vi "Delete Stale Samples.vi"(8 "error in (no error)":errorcluster, 11 "buffer":refnum<data-value>) -> (0 "error out":errorcluster, 1 "new channel length":i32, 2 "new buffer timestamp":timestamp format="%<%H:%M:%S%6u\n%x>T", 3 "buffer":refnum<data-value>)   [LabVIEW 2017, in "Waveforms (N Ch).lvclass"]
uses:
  <vilib>/addons/_NISVFA/_Shared subVIs/Data Objects/Waveforms (DBL)/Waveforms (N Ch).lvclass
  C:/Program Files (x86)/National Instruments/LabVIEW 2017/vi.lib/addons/_NISVFA/_Shared subVIs/Data Objects/Data/Data.lvclass
  <vilib>/addons/_NISVFA/_Shared subVIs/Data Objects/Data/Data.lvclass/Data.ctl
  <vilib>/addons/_NISVFA/_Shared subVIs/Data Objects/Waveforms (DBL)/Waveforms (N Ch).lvclass/Waveforms (N Ch).ctl
  <vilib>/addons/_NISVFA/_Shared subVIs/Common/svc_Get Waveform Subset (Index).vi
  <vilib>/addons/_NISVFA/_Shared subVIs/Common/sv_Get NI Property Name String.vi
  <vilib>/addons/_NISVFA/_Shared subVIs/Common/svc_Get Array Subset (Index).vi
  <vilib>/addons/_NISVFA/_Shared subVIs/Common/svc_Coerce Index and Length.vi
  <vilib>/addons/_NISVFA/_Shared subVIs/Common/svc_Conditional Merge Error.vi
  <vilib>/addons/_NISVFA/_Shared subVIs/Data Objects/Data/Data.lvclass
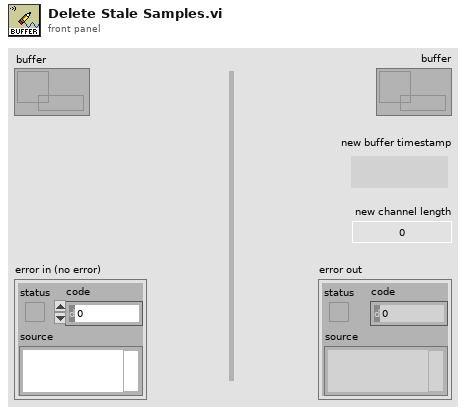
[diagram p1: front panel]
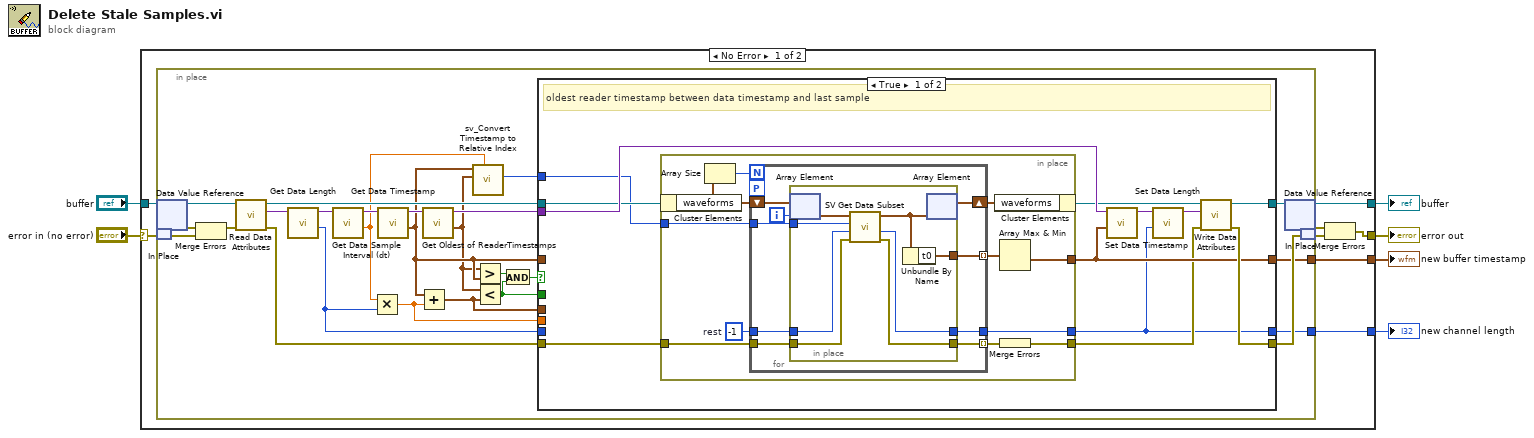
[diagram p0: block diagram]
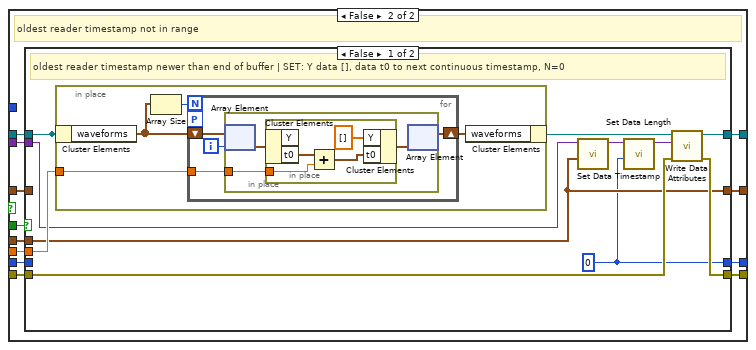
[diagram p2: hidden frame]
diagram:
  n1 = case shown="No Error" "error in (no error)" {
    selector: "error in (no error)" -> [w12 w122]
    tunnel: [w9 w122] -> w5
    tunnel: [w14 w123] -> w3
    tunnel: "buffer" -> [w13 w123]
    tunnel: [w8 _] -> w2
    tunnel: [w7 _] -> w1
    frame No Error {
      n2 = in-place {
        in-place-border: [w21] -> w8
        in-place-border: [w20] -> w7
        n3 = in-place-dvr #1(w13) -> (w39:refnum<class "Waveforms (N Ch).lvclass">, w38:errorcluster)
        n4 = in-place-match #2(w12) -> (w37:errorcluster)
        n5 = Merge Errors(w38, w37) -> (w36:errorcluster)
        n6 = call <vilib>:"Read Data Attributes.vi"("error in (no error)"=w36, "Data in"=w39) -> ("error out"=w34:errorcluster, "data attributes"=w28:variant, "Data out"=w35:refnum<class "Waveforms (N Ch).lvclass">)  [unwired: 7 in]
        n7 = call <vilib>:"Get Data Length.vi"("variant in"=w28) -> ("number of samples"=w19:i32, "variant out"=w29:variant)  [unwired: 9 in]
        n8 = call <vilib>:"Get Data Sample Interval (dt).vi"("variant in"=w29) -> ("dt [s]"=w18:dbl, "variant out"=w27:variant)  [unwired: 9 in]
        n9 = Multiply(x=w18, y=w19) -> (x*y=w22:dbl)
        n10 = call <vilib>:"Get Data Timestamp.vi"("variant in"=w27) -> ("timestamp"=w17:timestamp, "variant out"=w30:variant)  [unwired: 9 in]
        n11 = Add(x=w17, y=w22) -> (x+y=w23:timestamp)
        n12 = call <vilib>:"Get Oldest of ReaderTimestamps.vi"("data attributes"=w30) -> ("timestamp"=w16:timestamp, "data attributes"=w33:variant)  [unwired: 8 in, 1 out]
        n13 = call <vilib>:"sv_Convert Timestamp to Relative Index.vi"("waveform dt"=w18, "timestamp"=w16, "waveform timestamp"=w17) -> ("Y index"=w15:i32)  [unwired: 8 in]
        n14 = Greater?(x=w16, y=w17) -> (0:w25:bool)
        n15 = Less?(x=w16, y=w23) -> (x < y?=w24:bool)
        n16 = And(x=w25, y=w24) -> (x .and. y?=w26:bool)
        n17 = case shown="True" w26 {
          tunnel: w35 -> [w46 w88]
          tunnel: w34 -> [w43 w87]
          tunnel: w33 -> [w47 w91]
          tunnel: [w51 w90] -> w32
          tunnel: [w50 w89] -> w31
          tunnel: w24 -> [_ w86]
          tunnel: w23 -> [_ w85]
          tunnel: w22 -> [_ w84]
          tunnel: [w45 w83] -> w21
          tunnel: [w42 w82] -> w20
          tunnel: w17 -> [_ w81]
          tunnel: w19 -> [_ w80]
          tunnel: w15 -> [w40 _]
          frame True {
            # "oldest reader timestamp between data timestamp and last sample"
            n18 = in-place {
              in-place-border: w43 -> [w62]
              in-place-border: [w60] -> w45
              in-place-border: [w59] -> w44
              in-place-border: [w58] -> w42
              in-place-border: w40 -> [w56]
              w52 = -1  # rest
              n19 = in-place-cluster #3(w46) -> ("waveforms"=w53:waveform(dbl)[])
              n20 = Array Size(array=w53) -> (size(s)=w54:i32)
              n21 = for {
                N: w54 -> [_]
                tunnel: w62 -> [w71]
                tunnel: [w70] -> w57 mode=indexing
                tunnel: [w69] -> w61 mode=indexing
                workers-P: _ -> [_]
                tunnel: [w68] -> w58
                tunnel: w56 -> [w67]
                shift-right: [w64] -> w55
                shift-left: w53 -> [w66]
                tunnel: w52 -> [w63]
                i -> [w65]
                n22 = in-place {
                  in-place-border: w71 -> [w79]
                  in-place-border: [w78] -> w70
                  in-place-border: [w77] -> w69
                  in-place-border: [w76] -> w68
                  in-place-border: w67 -> [w75]
                  in-place-border: w63 -> [w72]
                  n23 = in-place-array #4(w66, w65) -> (w74:waveform(dbl))
                  n24 = call-poly <vilib>:"SV Get Data Subset.vi"("error in (no error)"=w79, "length (-1 = all)"=w72, "start index (0)"=w75, "waveform in"=w74) -> ("error out"=w78:errorcluster, "actual length"=w76:i32, "waveform subset"=w73:waveform(dbl))  [unwired: 2 in, 3 out]
                  n25 = Unbundle By Name(w73) -> ("t0"=w77:timestamp)
                  n26 = in-place-array #4(w73) -> (w64:waveform(dbl)[])  [unwired: 1 out]
                }
              }
              n27 = in-place-cluster #3("waveforms"=w55) -> (w41:refnum<class "Waveforms (N Ch).lvclass">)
              n28 = Array Max & Min(array=w61) -> (min value=w60:timestamp)  [unwired: 3 out]
              n29 = Merge Errors(w57) -> (w59:errorcluster)
            }
            n30 = call <vilib>:"Set Data Timestamp.vi"("timestamp"=w45, "variant in"=w47) -> ("variant out"=w49:variant)  [unwired: 9 in]
            n31 = call <vilib>:"Set Data Length.vi"("number of samples"=w42, "variant in"=w49) -> ("variant out"=w48:variant)  [unwired: 9 in]
            n32 = call <vilib>:"Write Data Attributes.vi"("error in (no error)"=w44, "data attributes"=w48, "Data in"=w41) -> ("error out"=w50:errorcluster, "Data out"=w51:refnum<class "Waveforms (N Ch).lvclass">)  [unwired: 7 in]
          }
          frame False {
            # "oldest reader timestamp not in range"
            n33 = case shown="False" w86 {
              tunnel: [w102 w121] -> w89
              tunnel: [w94 w120] -> _
              tunnel: [w101 w120] -> w90
              tunnel: w91 -> [w92 _]
              tunnel: w87 -> [w100 w121]
              tunnel: w88 -> [w94 w120]
              tunnel: w85 -> [w96 _]
              tunnel: w84 -> [w97 _]
              tunnel: [w96 w119] -> w83
              tunnel: [w95 w118] -> w82
              tunnel: w81 -> [_ w119]
              tunnel: w80 -> [_ w118]
              frame False {
                w95 = 0 ("number of samples")
                # "oldest reader timestamp newer than end of buffer | SET: Y data [], data t0 to next continuous timestamp, N=0"
                n34 = in-place {
                  in-place-border: w97 -> [w106]
                  n35 = in-place-cluster #5(w94) -> ("waveforms"=w103:waveform(dbl)[])
                  n36 = Array Size(array=w103) -> (size(s)=w104:i32)
                  n37 = for {
                    N: w104 -> [_]
                    tunnel: w106 -> [w110]
                    shift-right: [w107] -> w105
                    shift-left: w103 -> [w109]
                    workers-P: _ -> [_]
                    i -> [w108]
                    n38 = in-place {
                      in-place-border: w110 -> [w113]
                      n39 = in-place-array #6(w109, w108) -> (w112:waveform(dbl))
                      n40 = in-place {
                        in-place-border: w113 -> [w117]
                        n41 = in-place-cluster #7(w112) -> ("t0"=w116:timestamp)  [unwired: 1 out]
                        n42 = Add(x=w116, y=w117) -> (x+y=w115:timestamp)
                        n43 = in-place-cluster #7("Y"=dbl[] [], "t0"=w115) -> (w111:waveform(dbl))
                      }
                      n44 = in-place-array #6(w111) -> (w107:waveform(dbl)[])  [unwired: 1 out]
                    }
                  }
                  n45 = in-place-cluster #5("waveforms"=w105) -> (w93:refnum<class "Waveforms (N Ch).lvclass">)
                }
                n46 = call <vilib>:"Set Data Timestamp.vi"("timestamp"=w96, "variant in"=w92) -> ("variant out"=w99:variant)  [unwired: 9 in]
                n47 = call <vilib>:"Set Data Length.vi"("number of samples"=w95, "variant in"=w99) -> ("variant out"=w98:variant)  [unwired: 9 in]
                n48 = call <vilib>:"Write Data Attributes.vi"("error in (no error)"=w100, "data attributes"=w98, "Data in"=w93) -> ("error out"=w102:errorcluster, "Data out"=w101:refnum<class "Waveforms (N Ch).lvclass">)  [unwired: 7 in]
              }
              frame True {
                # "oldest reader timestamp older than data timestamp | NO Change to Buffer (expect Reader to fail next call unless reset = TRUE)"
              }
            }
          }
        }
        n49 = in-place-dvr #1(w32) -> (w14:refnum<data-value>, w11:errorcluster)
        n50 = in-place-match #2(w31) -> (w10:errorcluster)
      }
      n51 = Merge Errors(w11, w10) -> (w9:errorcluster)
    }
    frame Error {
    }
  }
  "error out" <- w5
  "buffer" <- w3
  "new channel length" <- w1
  "new buffer timestamp" <- w2
